vi "TLPM Get Resource Name2.vi"(8 "error in (no error)":errorcluster {"code" format="%.0x"}, 10 "Index (0)":u32) -> (0 "error out":errorcluster {"code" format="%.0x"}, 3 "instrument handle out":refnum<visa-resource-name>, 11 "Resource Name":string)   [LabVIEW 2023, in "Thorlabs Power Meter.lvlib"]
doc: "This VI gets the resource name string needed to open a device with <Initialize>.\n\nNotes:\n(1) The data provided by this VI was updated at the last call of <Find Resources>."
uses:
  Thorlabs Power Meter.lvlib
panel:
  in  "instrument handle":refnum<visa-resource-name>
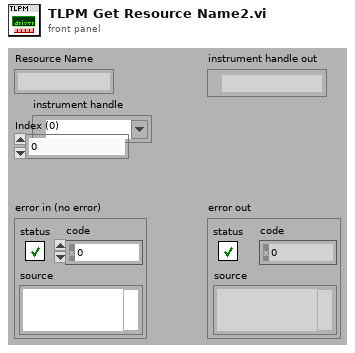
[diagram p1: front panel]
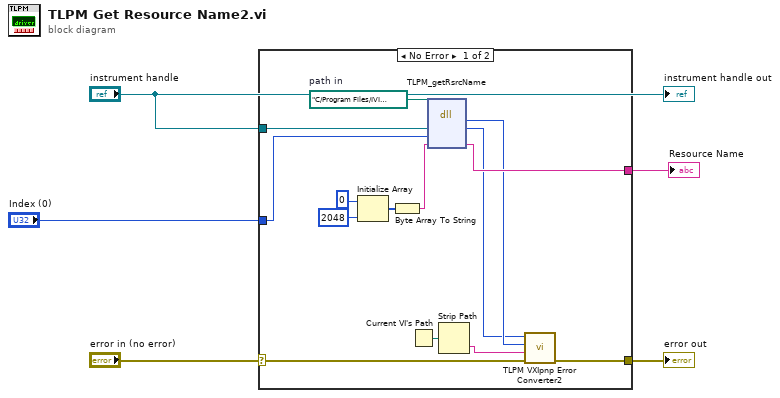
[diagram p0: block diagram]
diagram:
  n1 = case shown="No Error" "error in (no error)" {
    selector: "error in (no error)" -> [w10 w20]
    tunnel: [w11 w20] -> w5
    tunnel: "instrument handle" -> [w18 _]
    tunnel: "Index (0)" -> [w17 _]
    tunnel: [w12 _] -> w1
    frame No Error {
      w6 = path "C:/Program Files/IVI Foundation/VISA/Win64/Bin/TLPM_64.dll"  # path in
      n2 = Initialize Array(u8 0 ("element"), 2048 ("dimension size")) -> (w15:u8[])
      n3 = Byte Array To String(unsigned byte array=w15) -> (string=w16:string)
      n4 = Current VI's Path() -> (path=w19:path)
      n5 = dll-call lib="TLPM_64.dll" fn="TLPM_getRsrcName"(path in=w6, "Instrument Handle"=w18, "Index"=w17, "Resource Name"=w16) -> ("return type"=w8:i32, "Instrument Handle"=w7:u32, "Resource Name"=w12:string)  [unwired: 3 in, 2 out]
      n6 = Strip Path(path=w19) -> (name=w9:string)  [unwired: 1 out]
      n7 = call "TLPM VXIpnp Error Converter2.vi"("error in (no error)"=w10, "Name Of VI (\"\")"=w9, "CVI Error Code (0)"=w8, "instrument handle"=w7) -> ("error out"=w11:errorcluster)  [unwired: 6 in, 1 out]
    }
    frame Error {
    }
  }
  "error out" <- w5
  "Resource Name" <- w1
  "instrument handle out" <- "instrument handle"
